vi "Get DataType.vi"(8 "error in":errorcluster, 11 "Object Type in":refnum<class "Object Type Base.lvclass">) -> (0 "error out":errorcluster, 1 "Set?":bool, 2 "DataType":u16(ring) items=["UNKNOWN", "BOOLEAN", "INTEGER8", "INTEGER16", "INTEGER32", "UNSIGNED8", "UNSIGNED16", "UNSIGNED32", "REAL32", "VISIBLE_STRING", "OCTET_STRING", "UNICODE_STRING", "TIME_OF_DAY", "TIME_DIFFERENCE", "RESERVED1", "DOMAIN", "INTEGER24", "REAL64", "INTEGER40", "INTEGER48", "INTEGER56", "INTEGER64", "UNSIGNED24", "RESERVED2", "UNSIGNED40", "UNSIGNED48", "UNSIGNED56", "UNSIGNED64", "RESERVED3", "RESERVED4", "RESERVED5", "RESERVED6", "PDO_COMMUNICATION_PARAMETER", "PDO_MAPPING", "SDO_PARAMETER", "IDENTITY", "RESERVED7"], 3 "Object Type out":refnum<class "Object Type Base.lvclass">)   [LabVIEW 2019, in "Electronic Datasheet.lvlib" / "Object Type Base.lvclass"]
uses:
  Object Type Base.lvclass
  Object Type Base.lvclass/Object Type Base.ctl
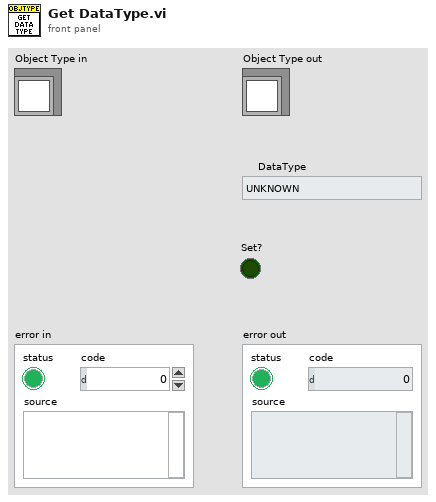
[diagram p1: front panel]
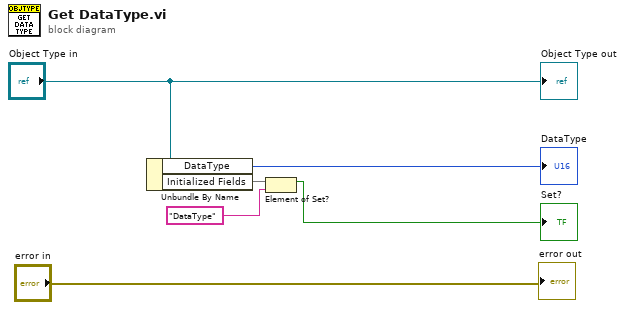
[diagram p0: block diagram]
diagram:
  n1 = Unbundle By Name("Object Type in") -> ("DataType"=→"DataType":u16, "Initialized Fields"=w4:set{string})
  n2 = Element of Set?(10:"DataType" ("element"), 11:w4) -> (3:→"Set?":bool)
  "Object Type out" <- "Object Type in"
  "error out" <- "error in"
